vi "GdsLanguage_GetLanguageData.vi"(5 "error in (no error)":errorcluster) -> (15 "Language":T1, 16 "StringIDArray":string[](array[string]), 17 "TranslatedStrings":string[](array[string]), 18 "FoundLanguages":T1[](array[typedef]), 19 "error out":errorcluster)   [LabVIEW 2016]
uses:
  <resource>/Framework/Providers/Open_GDS/ClassProviders/Common/GdsLanguage/GdsLanguage_LanguageID.ctl
  <resource>/Framework/Providers/Open_GDS/ClassProviders/Common/GdsLanguage/private/GdsLanguage_ChecksumCheckType.ctl
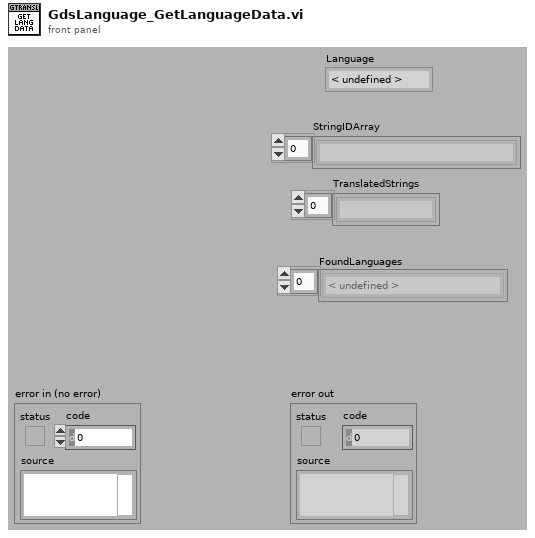
[diagram p1: front panel]
types:
  T1 = typedef "GdsLanguage_LanguageID.ctl" = enum16{"< undefined >", "aa", "ab", "af", "am", "ar", "as", "ay", "az", "ba", "be", "bg", "bh", "bi", "bn", "bo", "br", "ca", "co", "cs", "cy", "da", "de", "dz", "el", "en", "eo", "es", "et", "eu", "fa", "fi", "fj", "fo", "fr", "fy", "ga", "gd", "gl", "gn", "gu", "gv", "ha", "he", "hi", "hr", "hu", "hy", "ia", "id", "ie", "ik", "is", "it", "iu", "ja", "jv", "ka", "kk", "kl", "km", "kn", "ko", "ks", "ku", "ky", "la", "li", "ln", "lo", "lt", "lv", "mg", "mi", "mk", "ml", "mn", "mo", "mr", "ms", "mt", "my", "na", "ne", "nl", "no", "oc", "om", "or", "pa", "pl", "ps", "pt", "qu", "rm", "rn", "ro", "ru", "rw", "sa", "sd", "sg", "sh", "si", "sk", "sl", "sm", "sn", "so", "sq", "sr", "ss", "st", "su", "sv", "sw", "ta", "te", "tg", "th", "ti", "tk", "tl", "tn", "to", "tr", "ts", "tt", "tw", "ug", "uk", "ur", "uz", "vi", "vo", "wo", "xh", "yi", "yo", "zh", "zu"}
  T2 = typedef "GdsLanguage_ChecksumCheckType.ctl" = enum16{"NoControl", "CheckChecksum", "AddChecksum"}
  T3 = typedef "GdsLanguage_ObjectAttributes.ctl" = cluster{"Language":T1, "TranslatedStrings":string[], "StringIDArray":string[], "LanguageFilesDirectory":path, "AvailableLanguages":T1[]}
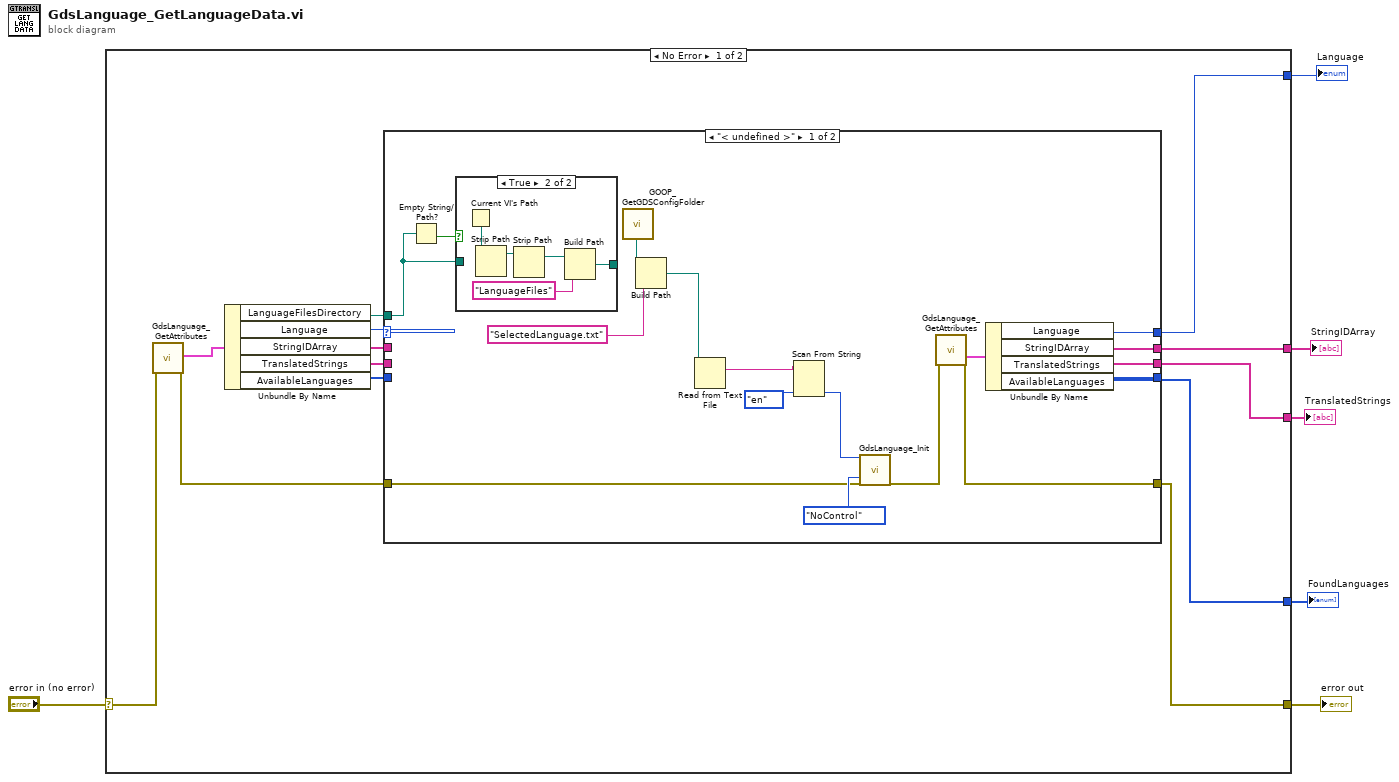
[diagram p0: block diagram]
diagram:
  n1 = case shown="No Error" "error in (no error)" {
    selector: "error in (no error)" -> [w18 w48]
    tunnel: [w7 w48] -> w5
    tunnel: [w14 _] -> w4
    tunnel: [w13 _] -> w3
    tunnel: [w16 _] -> w2
    tunnel: [w15 _] -> w1
    frame No Error {
      n2 = call <resource>:"GdsLanguage_GetAttributes.vi"("error in (no error)"=w18) -> ("Attributes"=w19:T3, "error out"=w9:errorcluster)  [unwired: 17 in]
      n3 = Unbundle By Name(w19) -> ("LanguageFilesDirectory"=w8:path, "Language"=w17:T1, "StringIDArray"=w12:string[], "TranslatedStrings"=w11:string[], "AvailableLanguages"=w10:T1[])
      n4 = case shown="\"< undefined >\"" w17 {
        selector: w17 -> [_ w47]
        tunnel: [w23 w47] -> w16
        tunnel: [w22 w46] -> w13
        tunnel: [w21 w45] -> w14
        tunnel: [w20 w44] -> w15
        tunnel: w12 -> [_ w46]
        tunnel: w11 -> [_ w45]
        tunnel: w10 -> [_ w44]
        tunnel: w9 -> [w32 w43]
        tunnel: w8 -> [w29 _]
        tunnel: [w24 w43] -> w7
        frame "< undefined >" {
          n5 = Empty String/Path?(string/path=w29) -> (empty?=w30:bool)
          n6 = case shown="True" w30 {
            tunnel: w29 -> [w37 _]
            tunnel: [w37 w39] -> _
            frame False {
            }
            frame True {
              n7 = Current VI's Path() -> (path=w38:path)
              n8 = Strip Path(path=w38) -> (stripped path=w42:path)  [unwired: 1 out]
              n9 = Strip Path(path=w42) -> (stripped path=w41:path)  [unwired: 1 out]
              n10 = Build Path(base path=w41, name or relative path="LanguageFiles") -> (appended path=w39:path)
            }
          }
          n11 = call <resource>:"GOOP_GetGDSConfigFolder.vi"() -> ("GDSFolderPath"=w31:path)
          n12 = Build Path(base path=w31, name or relative path="SelectedLanguage.txt") -> (appended path=w27:path)
          n13 = Read from Text File(file (use dialog)=w27) -> (text=w36:string)  [unwired: 3 in, 3 out]
          n14 = Scan From String(input string=w36, default 1=GdsLanguage_LanguageID."en" ("PrimaryLanguage")) -> (output 1=w34:T1)  [unwired: 3 in, 3 out]
          n15 = call <resource>:"GdsLanguage_Init.vi"("PrimaryLanguage"=w34, "ChesumControl"=GdsLanguage_ChecksumCheckType."NoControl", "error in (no error)"=w32) -> ("error out"=w25:errorcluster)  [unwired: 13 in, 3 out]
          n16 = call <resource>:"GdsLanguage_GetAttributes.vi"("error in (no error)"=w25) -> ("Attributes"=w26:T3, "error out"=w24:errorcluster)  [unwired: 17 in]
          n17 = Unbundle By Name(w26) -> ("Language"=w23:T1, "StringIDArray"=w22:string[], "TranslatedStrings"=w21:string[], "AvailableLanguages"=w20:T1[])
        }
        frame Default {
        }
      }
    }
    frame Error {
    }
  }
  "error out" <- w5
  "TranslatedStrings" <- w4
  "StringIDArray" <- w3
  "Language" <- w2
  "FoundLanguages" <- w1
